vi "Determine Digit Patterns.vi"(11 "Unique Patterns":string="acedgfb cdfbe gcdfa fbcad dab cefabd cdfgeb eafb cagedb ab") -> (3 "Digit Patterns":cluster{i32[]}[](array[cluster])=[{[0, 1, 2, 3, 4, 5]}, {[0, 1]}, {[0, 2, 3, 5, 6]}, {[0, 1, 2, 3, 5]}, {[0, 1, 4, 5]}, {[1, 2, 3, 4, 5]}, {[1, 2, 3, 4, 5, 6]}, {[0, 1, 3]}, {[0, 1, 2, 3, 4, 5, 6]}, {[0, 1, 2, 3, 4, 6]}])   [LabVIEW 2020]
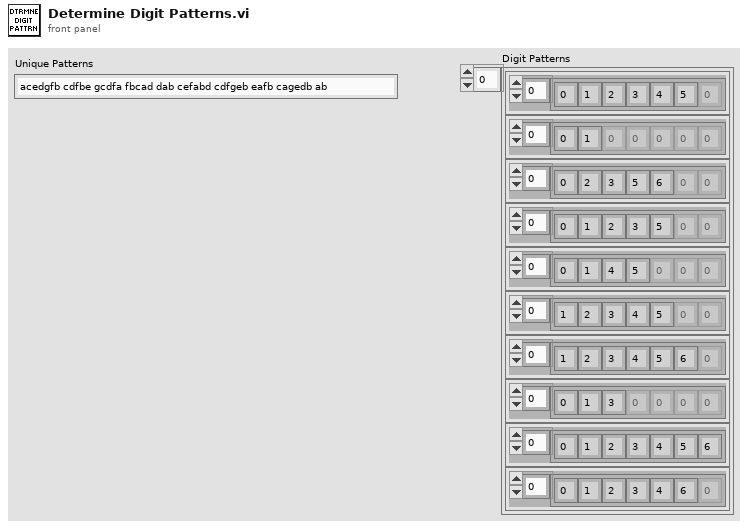
[diagram p1: front panel]
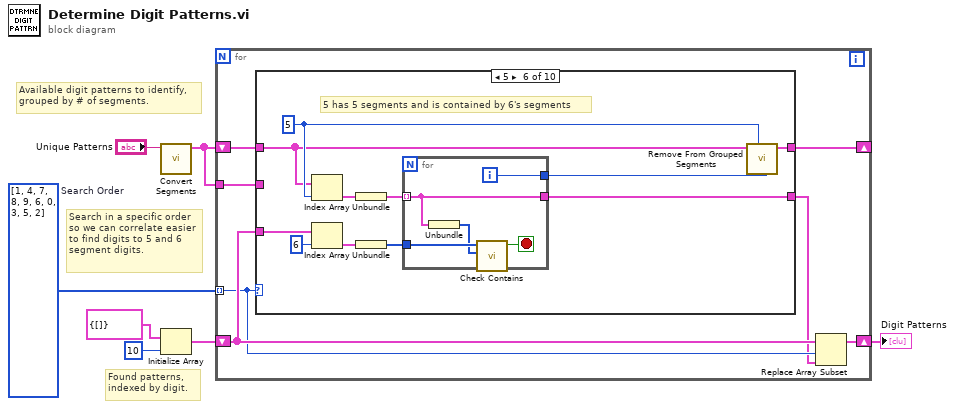
[diagram p0: block diagram]
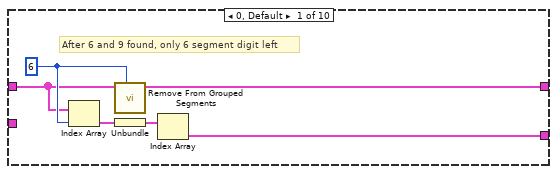
[diagram p2: hidden frame]
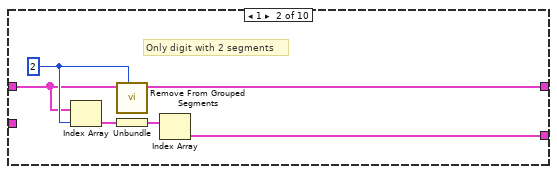
[diagram p3: hidden frame]
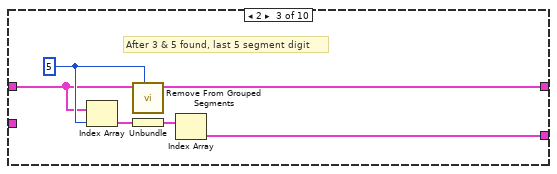
[diagram p4: hidden frame]
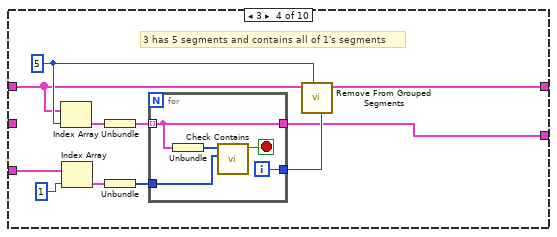
[diagram p5: hidden frame]
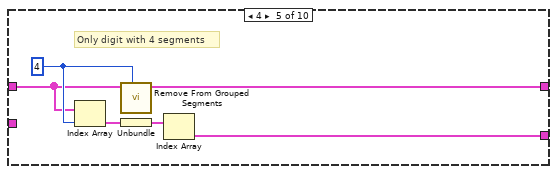
[diagram p6: hidden frame]
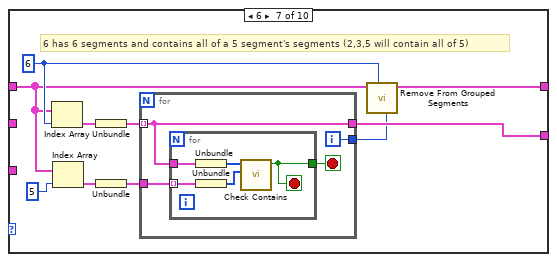
[diagram p7: hidden frame]
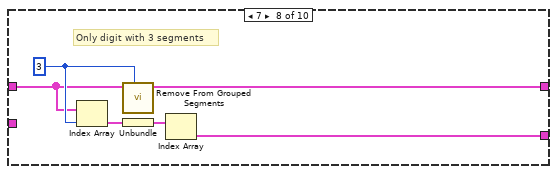
[diagram p8: hidden frame]
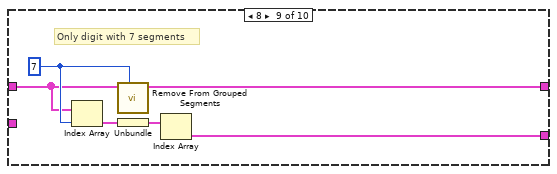
[diagram p9: hidden frame]
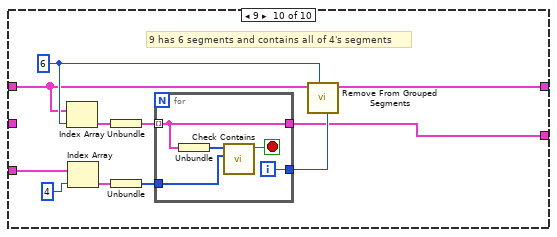
[diagram p10: hidden frame]
diagram:
  w2 = i32[] [1, 4, 7, 8, 9, 6, 0, 3, 5, 2]  # Search Order
  # "Search in a specific order so we can correlate easier to find digits to 5 and 6 segment digits."
  # "Available digit patterns to identify,\ngrouped by # of segments."
  # "Found patterns, indexed by digit."
  n1 = call "Convert Segments.vi"("Pattern String"="Unique Patterns") -> ("Length Grouped Segments"=w3:cluster{cluster{i32[]}[]}[])  [unwired: 9 in, 1 out]
  n2 = Initialize Array(cluster{i32[]} {[]}, 10 ("dimension size")) -> (w4:cluster{i32[]}[])
  n3 = for {
    shift-right: [w12] -> _
    shift-left: w3 -> [w14]
    tunnel: w3 -> [w13]
    tunnel: w2 -> [w9] mode=indexing
    shift-right: [w11] -> w1
    shift-left: w4 -> [w10]
    n4 = case shown="5" w9 {
      tunnel: w14 -> [w16 w23 w29 w36 w51 w63 w71 w92 w98 w105]
      tunnel: w13 -> [_ _ _ _ _ _ _ _ _ _]
      tunnel: [w15 w22 w28 w34 w50 w62 w72 w90 w97 w103] -> w12
      tunnel: w10 -> [_ _ _ w35 _ w60 _ _ _ w104]
      tunnel: [w18 w21 w27 w33 w49 w55 w75 w91 w96 w102] -> w8
      frame 0, Default {
        w17 = 6 ("index")
        # "After 6 and 9 found, only 6 segment digit left"
        n5 = Index Array(array=w16, index=w17) -> (element=w20:cluster{cluster{i32[]}[]})
        n6 = call "Remove From Grouped Segments.vi"("Length"=w17, "Length Grouped Segments In"=w16) -> ("Length Grouped Segments"=w15:cluster{cluster{i32[]}[]}[])  [unwired: 9 in]
        n7 = Unbundle(w20) -> (w19:cluster{i32[]}[])
        n8 = Index Array(array=w19) -> (element=w18:cluster{i32[]})  [unwired: 1 in]
      }
      frame 1 {
        w24 = 2 ("index")
        # "Only digit with 2 segments"
        n9 = Index Array(array=w23, index=w24) -> (element=w26:cluster{cluster{i32[]}[]})
        n10 = call "Remove From Grouped Segments.vi"("Length"=w24, "Length Grouped Segments In"=w23) -> ("Length Grouped Segments"=w22:cluster{cluster{i32[]}[]}[])  [unwired: 9 in]
        n11 = Unbundle(w26) -> (w25:cluster{i32[]}[])
        n12 = Index Array(array=w25) -> (element=w21:cluster{i32[]})  [unwired: 1 in]
      }
      frame 2 {
        w30 = 5 ("index")
        # "After 3 & 5 found, last 5 segment digit"
        n13 = Index Array(array=w29, index=w30) -> (element=w32:cluster{cluster{i32[]}[]})
        n14 = call "Remove From Grouped Segments.vi"("Length"=w30, "Length Grouped Segments In"=w29) -> ("Length Grouped Segments"=w28:cluster{cluster{i32[]}[]}[])  [unwired: 9 in]
        n15 = Unbundle(w32) -> (w31:cluster{i32[]}[])
        n16 = Index Array(array=w31) -> (element=w27:cluster{i32[]})  [unwired: 1 in]
      }
      frame 3 {
        w38 = 5
        # "3 has 5 segments and contains all of 1's segments"
        n17 = Index Array(array=w36, index=w38) -> (element=w40:cluster{cluster{i32[]}[]})
        n18 = Index Array(array=w35, index=1) -> (element=w42:cluster{i32[]})
        n19 = Unbundle(w40) -> (w39:cluster{i32[]}[])
        n20 = Unbundle(w42) -> (w41:i32[])
        n21 = for {
          tunnel: w41 -> [w47]
          tunnel: w39 -> [w44] mode=indexing
          tunnel: [w45] -> w37
          tunnel: [w44] -> w33
          i -> [w45]
          stop <- w46 stop-if-true
          n22 = Unbundle(w44) -> (w48:i32[])
          n23 = call "Check Contains.vi"("Segment B"=w47, "Segment A"=w48) -> ("A Contains B?"=w46:bool)  [unwired: 9 in]
        }
        n24 = call "Remove From Grouped Segments.vi"("Index"=w37, "Length"=w38, "Length Grouped Segments In"=w36) -> ("Length Grouped Segments"=w34:cluster{cluster{i32[]}[]}[])  [unwired: 8 in]
      }
      frame 4 {
        w52 = 4 ("index")
        # "Only digit with 4 segments"
        n25 = Index Array(array=w51, index=w52) -> (element=w54:cluster{cluster{i32[]}[]})
        n26 = call "Remove From Grouped Segments.vi"("Length"=w52, "Length Grouped Segments In"=w51) -> ("Length Grouped Segments"=w50:cluster{cluster{i32[]}[]}[])  [unwired: 9 in]
        n27 = Unbundle(w54) -> (w53:cluster{i32[]}[])
        n28 = Index Array(array=w53) -> (element=w49:cluster{i32[]})  [unwired: 1 in]
      }
      frame 5 {
        w64 = 5
        # "5 has 5 segments and is contained by 6's segments"
        n29 = Index Array(array=w63, index=w64) -> (element=w65:cluster{cluster{i32[]}[]})
        n30 = Index Array(array=w60, index=6) -> (element=w58:cluster{i32[]})
        n31 = Unbundle(w65) -> (w61:cluster{i32[]}[])
        n32 = Unbundle(w58) -> (w57:i32[])
        n33 = for {
          tunnel: w61 -> [w67] mode=indexing
          tunnel: w57 -> [w70]
          tunnel: [w68] -> w56
          tunnel: [w67] -> w55
          i -> [w68]
          stop <- w66 stop-if-true
          n34 = Unbundle(w67) -> (w69:i32[])
          n35 = call "Check Contains.vi"("Segment B"=w69, "Segment A"=w70) -> ("A Contains B?"=w66:bool)  [unwired: 9 in]
        }
        n36 = call "Remove From Grouped Segments.vi"("Index"=w56, "Length"=w64, "Length Grouped Segments In"=w63) -> ("Length Grouped Segments"=w62:cluster{cluster{i32[]}[]}[])  [unwired: 8 in]
      }
      frame 6 {
        w74 = 6
        # "6 has 6 segments and contains all of a 5 segment's segments (2,3,5 will contain all of 5)"
        n37 = Index Array(array=w71, index=w74) -> (element=w77:cluster{cluster{i32[]}[]})
        n38 = Index Array(array=w71, index=5) -> (element=w79:cluster{cluster{i32[]}[]})
        n39 = Unbundle(w77) -> (w76:cluster{i32[]}[])
        n40 = Unbundle(w79) -> (w78:cluster{i32[]}[])
        n41 = for {
          tunnel: w78 -> [w82]
          tunnel: w76 -> [w83] mode=indexing
          tunnel: [w84] -> w73
          tunnel: [w83] -> w75
          i -> [w84]
          stop <- w81 stop-if-true
          n42 = for {
            tunnel: w83 -> [w88]
            tunnel: w82 -> [w87] mode=indexing
            tunnel: [w85] -> w81
            stop <- w85 stop-if-true
            n43 = Unbundle(w88) -> (w89:i32[])
            n44 = Unbundle(w87) -> (w86:i32[])
            n45 = call "Check Contains.vi"("Segment B"=w86, "Segment A"=w89) -> ("A Contains B?"=w85:bool)  [unwired: 9 in]
          }
        }
        n46 = call "Remove From Grouped Segments.vi"("Index"=w73, "Length"=w74, "Length Grouped Segments In"=w71) -> ("Length Grouped Segments"=w72:cluster{cluster{i32[]}[]}[])  [unwired: 8 in]
      }
      frame 7 {
        w93 = 3 ("index")
        # "Only digit with 3 segments"
        n47 = Index Array(array=w92, index=w93) -> (element=w95:cluster{cluster{i32[]}[]})
        n48 = call "Remove From Grouped Segments.vi"("Length"=w93, "Length Grouped Segments In"=w92) -> ("Length Grouped Segments"=w90:cluster{cluster{i32[]}[]}[])  [unwired: 9 in]
        n49 = Unbundle(w95) -> (w94:cluster{i32[]}[])
        n50 = Index Array(array=w94) -> (element=w91:cluster{i32[]})  [unwired: 1 in]
      }
      frame 8 {
        w99 = 7 ("index")
        # "Only digit with 7 segments"
        n51 = Index Array(array=w98, index=w99) -> (element=w101:cluster{cluster{i32[]}[]})
        n52 = call "Remove From Grouped Segments.vi"("Length"=w99, "Length Grouped Segments In"=w98) -> ("Length Grouped Segments"=w97:cluster{cluster{i32[]}[]}[])  [unwired: 9 in]
        n53 = Unbundle(w101) -> (w100:cluster{i32[]}[])
        n54 = Index Array(array=w100) -> (element=w96:cluster{i32[]})  [unwired: 1 in]
      }
      frame 9 {
        w107 = 6
        # "9 has 6 segments and contains all of 4's segments"
        n55 = Index Array(array=w105, index=w107) -> (element=w109:cluster{cluster{i32[]}[]})
        n56 = Index Array(array=w104, index=4) -> (element=w111:cluster{i32[]})
        n57 = Unbundle(w109) -> (w108:cluster{i32[]}[])
        n58 = Unbundle(w111) -> (w110:i32[])
        n59 = for {
          tunnel: w110 -> [w116]
          tunnel: w108 -> [w113] mode=indexing
          tunnel: [w114] -> w106
          tunnel: [w113] -> w102
          i -> [w114]
          stop <- w115 stop-if-true
          n60 = Unbundle(w113) -> (w117:i32[])
          n61 = call "Check Contains.vi"("Segment B"=w116, "Segment A"=w117) -> ("A Contains B?"=w115:bool)  [unwired: 9 in]
        }
        n62 = call "Remove From Grouped Segments.vi"("Index"=w106, "Length"=w107, "Length Grouped Segments In"=w105) -> ("Length Grouped Segments"=w103:cluster{cluster{i32[]}[]}[])  [unwired: 8 in]
      }
    }
    n63 = Replace Array Subset(array=w10, new element=w8, index=w9) -> (w11:cluster{i32[]}[])
  }
  "Digit Patterns" <- w1
